vi "turn_rate_to_left_motor.vi"(1 "Turn Rate":dbl) -> (0 "Left Voltage":dbl step=0.01)   [LabVIEW 2009]
uses:
  <vilib>/gmath/NI_Gmath.lvlib
panel:
  in  "Left Voltage / turn rate":cluster{"voltage":dbl, "turn rate":dbl}[](array[cluster])=[{"voltage"=0.0833, "turn rate"=-120.5}, {"voltage"=0.5536, "turn rate"=-119.8}, {"voltage"=1.0586, "turn rate"=-100.6}, {"voltage"=1.5647, "turn rate"=-76.36}, {"voltage"=2.0625, "turn rate"=-40.02}, {"voltage"=2.5, "turn rate"=0.0}, {"voltage"=3.0556, "turn rate"=38.01}, {"voltage"=3.5893, "turn rate"=73.52}, {"voltage"=4.0887, "turn rate"=99.54}, {"voltage"=5.0, "turn rate"=118.4}]
  # "Voltage is in V\nThrust in deg/s"
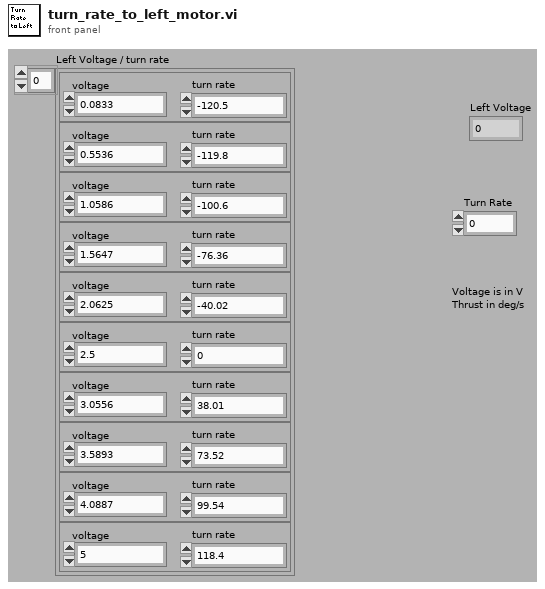
[diagram p1: front panel]
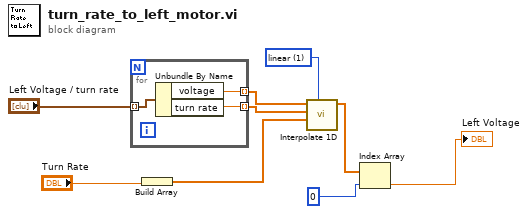
[diagram p0: block diagram]
diagram:
  w6 = 1 items=["nearest", "linear", "spline", "cubic Hermite", "Lagrange"] ("method")
  n1 = for {
    tunnel: "Left Voltage / turn rate" -> [w12] mode=indexing
    tunnel: [w11] -> w8 mode=indexing
    tunnel: [w10] -> w7 mode=indexing
    n2 = Unbundle By Name(w12) -> ("voltage"=w11:dbl, "turn rate"=w10:dbl)
  }
  n3 = Build Array("Turn Rate") -> (w5:dbl[])
  n4 = call <vilib>:"Interpolate 1D.vi"("method"=w6, "xi"=w5, "X"=w7, "Y"=w8) -> ("yi"=w3:dbl[])  [unwired: 5 in, 2 out]
  n5 = Index Array(array=w3, index=0) -> (element=→"Left Voltage":dbl)
